vi "arduino_close_subIV.vi"(9 "arduino 1-6 addresses and errors out":T1, 11 "arduinos on?":bool) -> ()   [LabVIEW 2014]
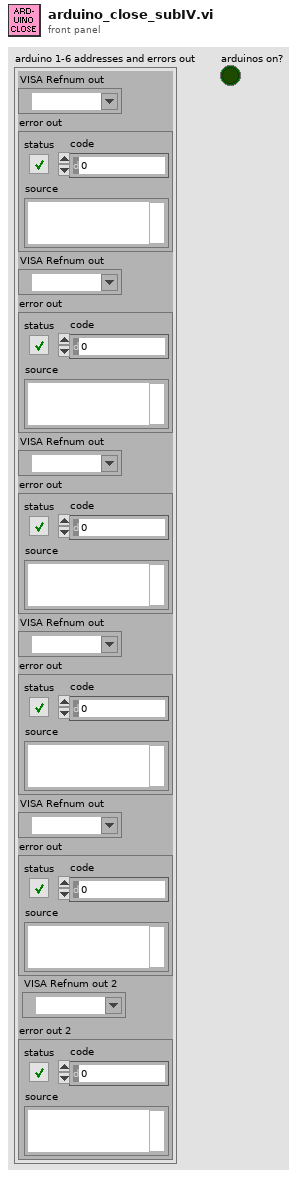
[diagram p1: front panel]
types:
  T1 = cluster{"VISA Refnum out":refnum<visa-resource-name>, "error out":errorcluster, "VISA Refnum out":refnum<visa-resource-name>, "error out":errorcluster, "VISA Refnum out":refnum<visa-resource-name>, "error out":errorcluster, "VISA Refnum out":refnum<visa-resource-name>, "error out":errorcluster, "VISA Refnum out":refnum<visa-resource-name>, "error out":errorcluster, "VISA Refnum out 2":refnum<visa-resource-name>, "error out 2":errorcluster}
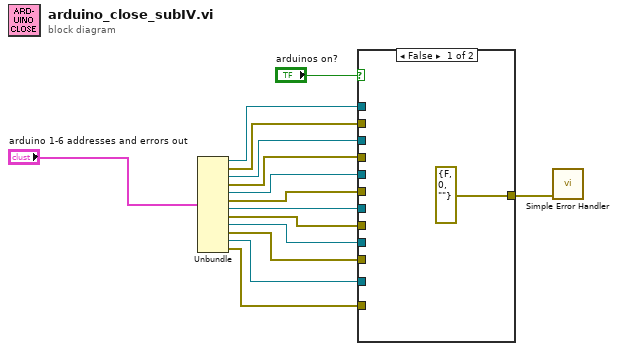
[diagram p0: block diagram]
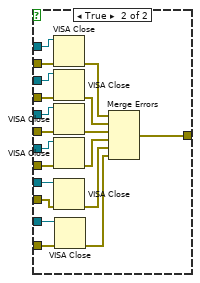
[diagram p2: hidden frame]
diagram:
  n1 = Unbundle("arduino 1-6 addresses and errors out") -> ("VISA Refnum out"=w13:refnum<visa-resource-name>, "error out"=w12:errorcluster, "VISA Refnum out"=w11:refnum<visa-resource-name>, "error out"=w4:errorcluster, "VISA Refnum out"=w5:refnum<visa-resource-name>, "error out"=w6:errorcluster, "VISA Refnum out"=w7:refnum<visa-resource-name>, "error out"=w8:errorcluster, "VISA Refnum out"=w9:refnum<visa-resource-name>, "error out"=w10:errorcluster, "VISA Refnum out 2"=w3:refnum<visa-resource-name>, "error out 2"=w2:errorcluster)
  n2 = case shown="False" "arduinos on?" {
    tunnel: w13 -> [_ w30]
    tunnel: w12 -> [_ w29]
    tunnel: w11 -> [_ w28]
    tunnel: w4 -> [_ w27]
    tunnel: w5 -> [_ w26]
    tunnel: w6 -> [_ w25]
    tunnel: w7 -> [_ w24]
    tunnel: w8 -> [_ w23]
    tunnel: w9 -> [_ w22]
    tunnel: w10 -> [_ w21]
    tunnel: w3 -> [_ w19]
    tunnel: w2 -> [_ w18]
    tunnel: [errorcluster {"status"=FALSE, "code"=0, "source"=""} ("error in (no error)") w17] -> w1
    frame False {
    }
    frame True {
      n3 = VISA Close(VISA resource name=w30, error in (no error)=w29) -> (error out=w35:errorcluster)
      n4 = VISA Close(VISA resource name=w28, error in (no error)=w27) -> (error out=w34:errorcluster)
      n5 = VISA Close(VISA resource name=w26, error in (no error)=w25) -> (error out=w33:errorcluster)
      n6 = VISA Close(VISA resource name=w24, error in (no error)=w23) -> (error out=w32:errorcluster)
      n7 = VISA Close(VISA resource name=w22, error in (no error)=w21) -> (error out=w31:errorcluster)
      n8 = VISA Close(VISA resource name=w19, error in (no error)=w18) -> (error out=w20:errorcluster)
      n9 = Merge Errors(w35, w34, w33, w32, w31, w20) -> (w17:errorcluster)
    }
  }
  n10 = call <vilib>:"Simple Error Handler.vi"("error in (no error)"=w1) -> ()  [unwired: 4 in, 5 out]
